vi "VLC - LabVIEW Embedded.vi"(5 "Media Source":string="dshow:// vdev=\"cam0\" adev=\"cam0\"", 7 "Script":string, 11 "error in (no error)":errorcluster) -> (15 "error out":errorcluster)   [LabVIEW 2011]
uses:
  Program Files (x86)/VideoLAN/VLC/libvlc.dll
  user32.dll
panel:
  # "http://www.videolan.org/developers/vlc/doc/doxygen/html/modules.html"
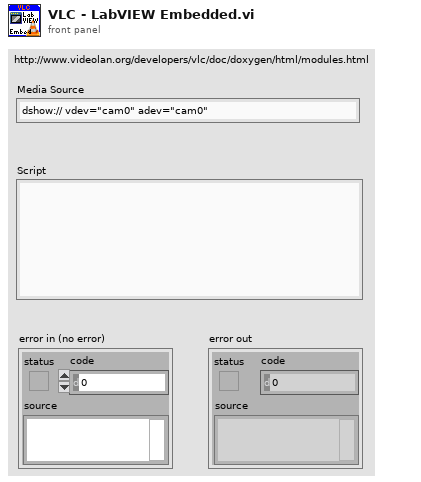
[diagram p1: front panel]
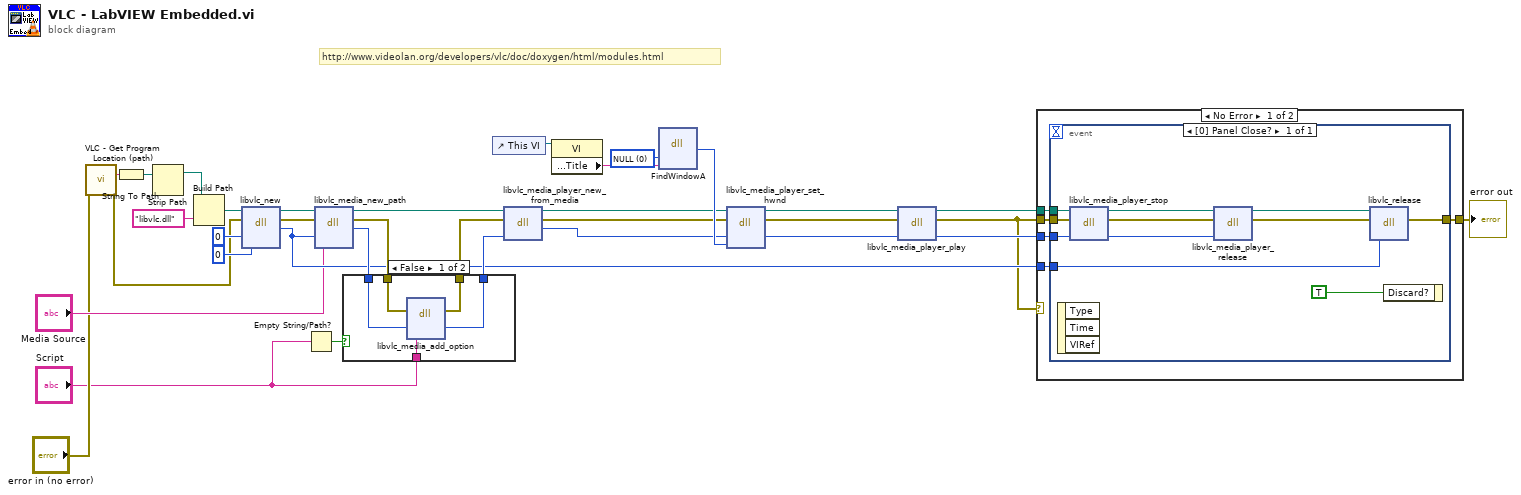
[diagram p0: block diagram]
diagram:
  w21 = 0 items=["NULL"]
  # "http://www.videolan.org/developers/vlc/doc/doxygen/html/modules.html"
  n1 = call "VLC - Get Program Location (path).vi"("error in (no error)"="error in (no error)") -> ("VLC path"=w12:string, "error out"=w5:errorcluster)  [unwired: 13 in]
  n2 = String To Path(string=w12) -> (path=w11:path)
  n3 = Strip Path(path=w11) -> (stripped path=w10:path)  [unwired: 1 out]
  n4 = Build Path(base path=w10, name or relative path="libvlc.dll") -> (appended path=w8:path)
  n5 = dll-call lib="C:/Program Files (x86)/VideoLAN/VLC/libvlc.dll" fn="libvlc_new"(path in=w8, error in=w5, "argc"=i16 0, "argv"=u8 0) -> (path out=w17:path, error out=w23:errorcluster, "return type"=w30:i32)  [unwired: 3 in]
  n6 = Empty String/Path?(string/path="Script") -> (empty?=w3:bool)
  n7 = dll-call lib="C:/Program Files (x86)/VideoLAN/VLC/libvlc.dll" fn="libvlc_media_new_path"(path in=w17, error in=w23, "p_instance"=w30, "path"="Media Source") -> (path out=w16:path, error out=w31:errorcluster, "return type"=w32:i32)  [unwired: 3 in]
  n8 = case shown="False" w3 {
    tunnel: w31 -> [w39 w41]
    tunnel: w32 -> [w38 w40]
    tunnel: [w37 w40] -> w33
    tunnel: [w36 w41] -> w34
    tunnel: "Script" -> [w35 _]
    frame False {
      n9 = dll-call lib="C:/Program Files (x86)/VideoLAN/VLC/libvlc.dll" fn="libvlc_media_add_option"(error in=w39, "p_md"=w38, "ppsz_options"=w35) -> (error out=w36:errorcluster, "p_md"=w37:i32)  [unwired: 4 in, 1 out]
    }
    frame True {
    }
  }
  n10 = control-ref of="This VI"() -> (w22:refnum<vi>)
  n11 = dll-call lib="C:/Program Files (x86)/VideoLAN/VLC/libvlc.dll" fn="libvlc_media_player_new_from_media"(path in=w16, error in=w34, "p_md"=w33) -> (path out=w15:path, error out=w26:errorcluster, "return type"=w24:i32)  [unwired: 2 in]
  n12 = property class="VI"(reference=w22) -> ("Front Panel.Title"=w20:string)  [unwired: 1 in, 2 out]
  n13 = dll-call lib="USER32.DLL" fn="FindWindowA" label="FindWindow"("lpszClassName"=w21, "lpszWindowName"=w20) -> ("hWnd"=w28:u32)  [unwired: 5 in, 2 out]
  n14 = dll-call lib="C:/Program Files (x86)/VideoLAN/VLC/libvlc.dll" fn="libvlc_media_player_set_hwnd"(path in=w15, error in=w26, "p_mi"=w24, "drawable"=w28) -> (path out=w14:path, error out=w27:errorcluster, "p_mi"=w25:i32)  [unwired: 3 in]
  n15 = dll-call lib="C:/Program Files (x86)/VideoLAN/VLC/libvlc.dll" fn="libvlc_media_player_play"(path in=w14, error in=w27, "p_mi"=w25) -> (path out=w13:path, error out=w1:errorcluster, "p_mi"=w29:i32)  [unwired: 2 in]
  n16 = case shown="No Error" w1 {
    tunnel: w30 -> [w46 _]
    tunnel: w29 -> [w45 _]
    tunnel: w1 -> [w44 w58]
    tunnel: w13 -> [w43 _]
    tunnel: [w42 w58] -> w2
    frame No Error {
      n17 = event shown="[0] Panel Close?" {
        selector: _ -> [_]
        dyn-events: _ -> [_]
        timeout: _ -> [_]
        tunnel: w44 -> [w57]
        tunnel: w45 -> [w56]
        tunnel: w46 -> [w52]
        tunnel: w43 -> [w50]
        tunnel: [w47] -> w42
        event Panel Close? {
          n18 = event-data() -> ()  [unwired: 1 in, 3 out]
          n19 = dll-call lib="C:/Program Files (x86)/VideoLAN/VLC/libvlc.dll" fn="libvlc_media_player_stop"(path in=w50, error in=w57, "p_mi"=w56) -> (path out=w49:path, error out=w55:errorcluster, "p_mi"=w54:i32)  [unwired: 2 in]
          n20 = dll-call lib="C:/Program Files (x86)/VideoLAN/VLC/libvlc.dll" fn="libvlc_media_player_release"(path in=w49, error in=w55, "p_mi"=w54) -> (path out=w48:path, error out=w53:errorcluster)  [unwired: 3 in]
          n21 = dll-call lib="C:/Program Files (x86)/VideoLAN/VLC/libvlc.dll" fn="libvlc_release"(path in=w48, error in=w53, "p_instnace"=w52) -> (error out=w47:errorcluster)  [unwired: 3 in, 1 out]
          n22 = event-data("Discard?"=TRUE) -> ()  [unwired: 1 in, 1 out]
        }
      }
    }
    frame Error {
    }
  }
  "error out" <- w2
